vi "Detect and Decode Multiple (Greyscale).vi"(8 "error in (no error)":errorcluster, 10 "Greyscale Image in":T4, 11 "WeChat QR Code Detector in":refnum<class "WeChat QR Code Detector.lvclass">) -> (0 "error out":errorcluster, 2 "Detections":T1[](array[typedef]), 3 "WeChat QR Code Detector":refnum<class "WeChat QR Code Detector.lvclass">)   [LabVIEW 2020, in "feature_detection.lvlib" / "WeChat QR Code Detector.lvclass"]
doc: "Detec and Decode Multiple QR Codes in the Image."
uses:
  WeChat QR Code Detector.lvclass
  image/Greyscale Image.ctl
  Detection.ctl
  common/Image Points Quad (Float).ctl
  common/Image Point (Float).ctl
  WeChat QR Code Detector.lvclass/WeChat QR Code Detector.ctl
  de44e2b3-a41c-416e-9770-09f180cbffa1.vi
  <vilib>/Utility/error.llb/Error Cluster From Error Code.vi
  common/common.lvlib
  image/image.lvlib
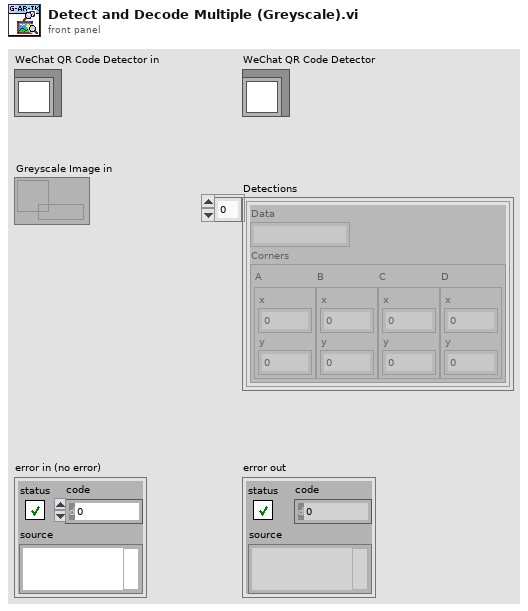
[diagram p1: front panel]
types:
  T1 = typedef "feature_detection.lvlib/WeChat QR Code Detector.lvclass/Detection.ctl" = cluster{"Data":string, "Corners":T2}
  T2 = typedef "common.lvlib/Image Points Quad (Float).ctl" = cluster{"A":T3, "B":T3, "C":T3, "D":T3}
  T3 = typedef "common.lvlib/Image Point (Float).ctl" = cluster{"x":dbl, "y":dbl}
  T4 = typedef "image.lvlib/Greyscale Image.ctl" = refnum<data-value>
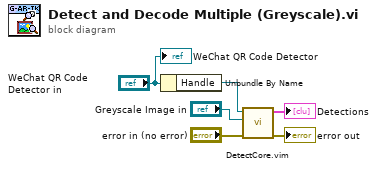
[diagram p0: block diagram]
diagram:
  n1 = Unbundle By Name("WeChat QR Code Detector in") -> ("Handle"=w1:refnum<data-value>)
  n2 = call "DetectCore.vim"("error in (no error)"="error in (no error)", "Greyscale Image"="Greyscale Image in", "Handle"=w1) -> ("error out"=→"error out":errorcluster, "Detections"=→"Detections":T1[])  [unwired: 7 in]
  "WeChat QR Code Detector" <- "WeChat QR Code Detector in"
